vi "NFL_L_bank_Control_09.vi"(0 "SI804.lvclass in":refnum<class "SI804.lvclass">, 7 "3 JSA20 DT118\nXA01":bool, 11 "error in":errorcluster) -> (4 "SI804.lvclass out":refnum<class "SI804.lvclass">, 8 "NFL L withdr":bool, 15 "error out":errorcluster)   [LabVIEW 2022 SP3, in "SI804.lvclass"]
uses:
  SI804.lvclass
  SI804.lvclass/SI804.ctl
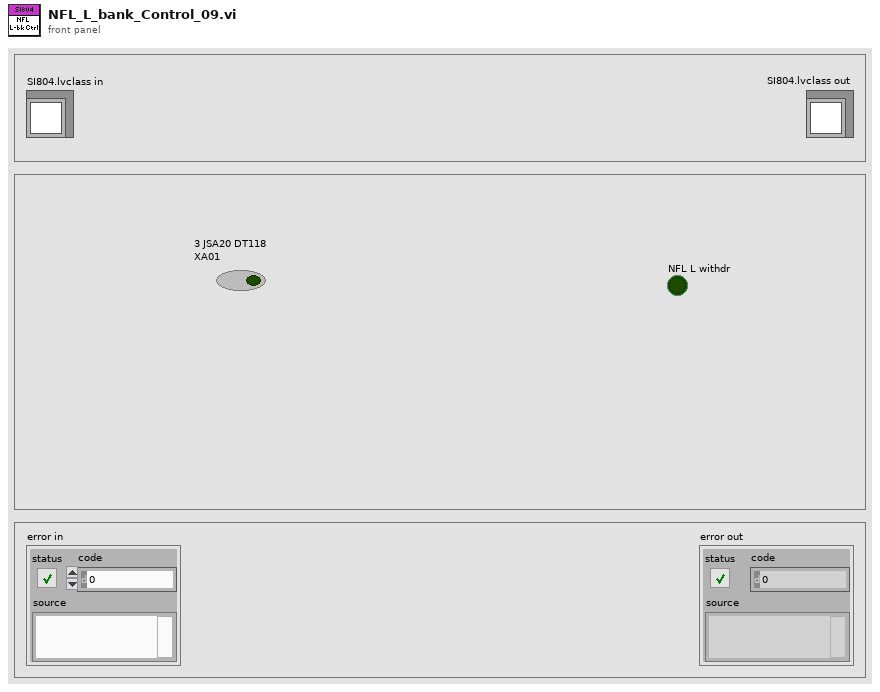
[diagram p1: front panel]
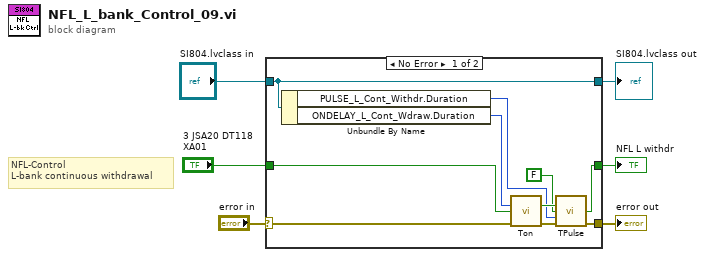
[diagram p0: block diagram]
diagram:
  # "NFL-Control\nL-bank continuous withdrawal"
  n1 = case shown="No Error" "error in" {
    selector: "error in" -> [w15 w17]
    tunnel: "3 JSA20 DT118\nXA01" -> [w16 _]
    tunnel: [w12 _] -> w4
    tunnel: "SI804.lvclass in" -> [w7 w18]
    tunnel: [w8 w17] -> w1
    tunnel: [w7 w18] -> w2
    frame No Error {
      n2 = Unbundle By Name(w7) -> ("PULSE_L_Cont_Withdr.Duration"=w10:i32, "ONDELAY_L_Cont_Wdraw.Duration"=w11:i32)
      n3 = call "Ton.vi"("Ton"=w11, "input"=w16, "error in"=w15) -> ("Pulse"=w13:bool, "error out"=w14:errorcluster)  [unwired: 8 in, 3 out]
      n4 = call "TPulse.vi"("trigger"=w13, "Reset"=FALSE, "TPulse"=w10, "error in"=w14) -> ("output"=w12:bool, "error out"=w8:errorcluster)  [unwired: 9 in, 1 out]
    }
    frame Error {
    }
  }
  "NFL L withdr" <- w4
  "SI804.lvclass out" <- w2
  "error out" <- w1
